vi "xio.newdir_lua.vi"(5 "LuaVIEW reference":T1) -> (15 "error out":errorcluster)   [LabVIEW 2012]
doc: "Creates a new directory.\nParameters:\nstr:path path of the directory to create.\nErrors:\nParent directory does not exist.\nFile or directory already exists at the specified path.\nDisk full."
uses:
  typedefs/t_LuaVIEW Reference.ctl
  subvis/private/LuaVIEW Pull (path).vi
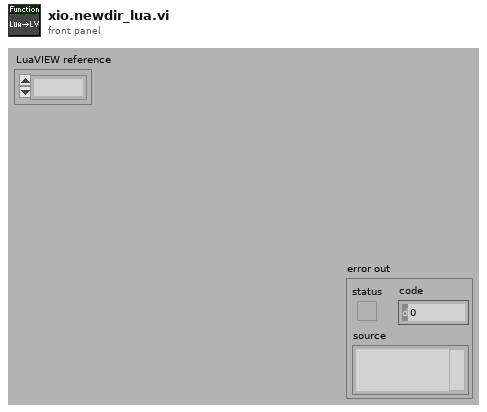
[diagram p1: front panel]
types:
  T1 = typedef "t_LuaVIEW Reference.ctl" = refnum<k1>
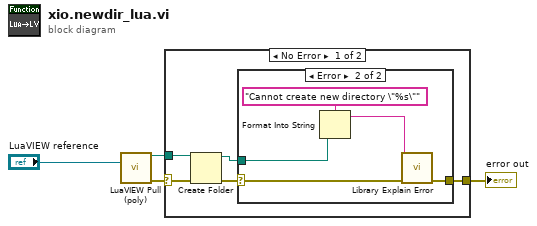
[diagram p0: block diagram]
diagram:
  n1 = call-poly "LuaVIEW Pull (poly).vi"("LuaVIEW reference in"="LuaVIEW reference") -> ("path"=w2:path, "error out"=w3:errorcluster)  [unwired: 12 in, 1 out]
  n2 = case shown="No Error" w3 {
    selector: w3 -> [w9 w16]
    tunnel: [w7 w16] -> w1
    tunnel: w2 -> [w6 _]
    frame No Error {
      n3 = Create Folder(path (use dialog)=w6, error in=w9) -> (created path=w5:path, error out=w8:errorcluster)  [unwired: 1 in, 1 out]
      n4 = case shown="Error" w8 {
        selector: w8 -> [w10 w15]
        tunnel: [w10 w14] -> w7
        tunnel: w5 -> [_ w11]
        frame No Error {
        }
        frame Error {
          n5 = Format Into String(format string="Cannot create new directory \"%s\"", w11) -> (resulting string=w13:string)  [unwired: 2 in, 1 out]
          n6 = call "Library Explain Error.vi"("explanation prefix (none)"=w13, "error in (no error)"=w15) -> ("explained error"=w14:errorcluster)  [unwired: 13 in]
        }
      }
    }
    frame Error {
    }
  }
  "error out" <- w1
